vi "G4SubTemplate_Singleton_4x4x4_CleanUp.vi"(8 "error in (no error)":errorcluster) -> (0 "error out":errorcluster)   [LabVIEW 2020, in "G4SubTemplate_Singleton_4x4x4.lvclass"]
uses:
  <resource>/Framework/Providers/Open_GDS/ClassProviders/Provider_EndevoGOOP400/Templates/G4SubTemplate_Singleton_4x4x4/G4SubTemplate_Singleton_4x4x4.lvclass
  <resource>/Framework/Providers/Open_GDS/ClassProviders/Provider_EndevoGOOP400/Templates/G4BaseTemplate_Singleton_4x4x4/G4BaseTemplate_Singleton_4x4x4.lvclass
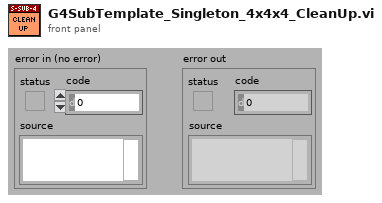
[diagram p1: front panel]
types:
  T1 = typedef "G4SubTemplate_Singleton_4x4x4.lvclass/ObjectAttributes.ctl" = cluster{"Attribute1":dbl}
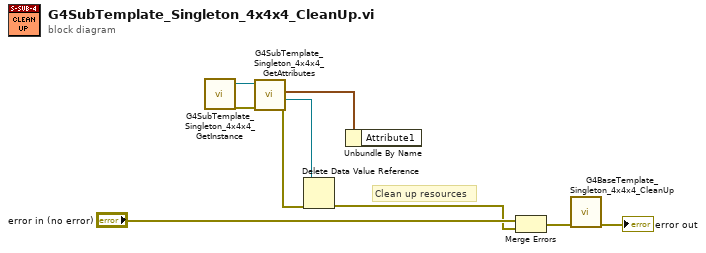
[diagram p0: block diagram]
diagram:
  # "Clean up resources"
  n1 = call <resource>:"G4SubTemplate_Singleton_4x4x4_GetInstance.vi"() -> ("error out"=w8:errorcluster, "reference out"=w7:refnum<class "G4SubTemplate_Singleton_4x4x4.lvclass">)  [unwired: 7 in, 3 out]
  n2 = call <resource>:"G4SubTemplate_Singleton_4x4x4_GetAttributes.vi"("error in (no error)"=w8, "reference in"=w7) -> ("error out"=w4:errorcluster, "DataRef"=w3:refnum<data-value>, "Data"=w9:T1)  [unwired: 6 in, 1 out]
  n3 = Delete Data Value Reference(data value reference=w3, error in=w4) -> (error out=w1:errorcluster)  [unwired: 1 out]
  n4 = Unbundle By Name(w9) -> ()  [unwired: 1 out]
  n5 = Merge Errors("error in (no error)", w1) -> (w6:errorcluster)
  n6 = call <resource>:"G4BaseTemplate_Singleton_4x4x4_CleanUp.vi"("error in (no error)"=w6) -> ("error out"=→"error out":errorcluster)  [unwired: 10 in]
